vi "Initialization Error Status.vi"(8 "error in (no error)":errorcluster, 11 "Node Ptr":T1 format="%.0x") -> (0 "error out":errorcluster)   [LabVIEW 2015, in "DMM-SWITCH-ScanList System Explorer.lvlib"]
uses:
  DMM-SWITCH-ScanList System Explorer.lvlib
  <vilib>/NI Veristand/Custom Device API/Custom Device Item Ref.ctl
  <vilib>/NI Veristand/Custom Device API/Custom Device API.lvlib
panel:
  out "Channel Settings":i32(listbox)
  in  "Header":cluster{"Section Name":string}={"Section Name"="Custom Device Item Settings"}
  in  "Description":string
  in  "Name":string
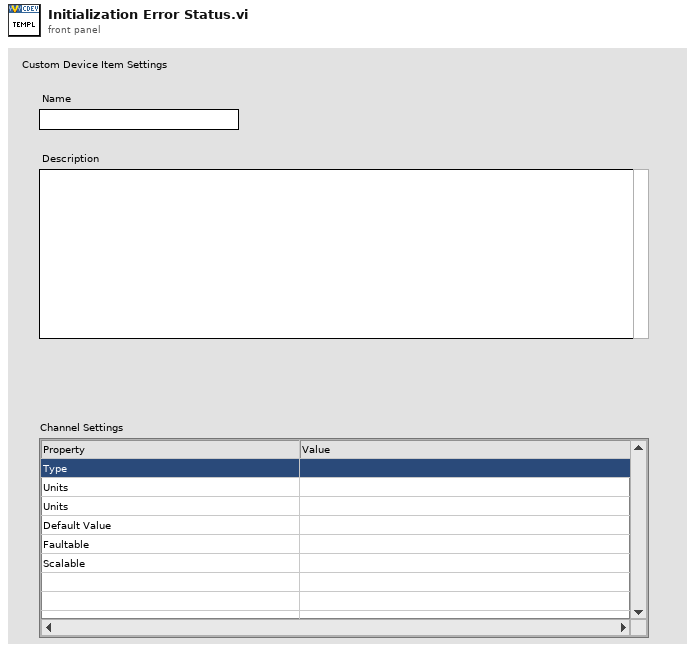
[diagram p1: front panel]
types:
  T1 = typedef "Custom Device API.lvlib/Custom Device Item Ref.ctl" = u64
  T2 = typedef "Custom Device API.lvlib/Custom Device Item Info.ctl" = cluster{"Name":string, "Is Channel":bool, "GUID":string, "Is Waveform":bool}
  T3 = typedef "Custom Device API.lvlib/Custom Device Commands.ctl" = enum16{"Default", "Item renamed", "Shutdown", "Dynamic button pressed"}
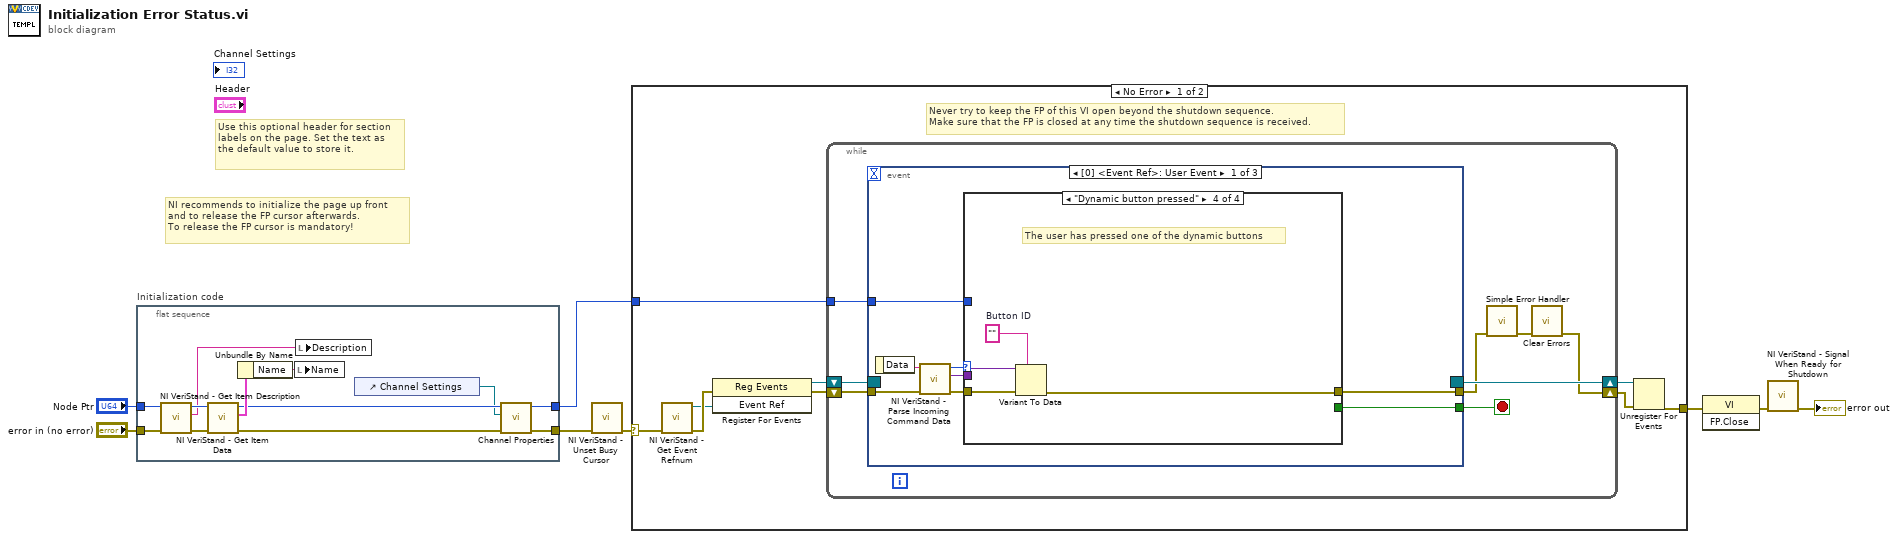
[diagram p0: block diagram]
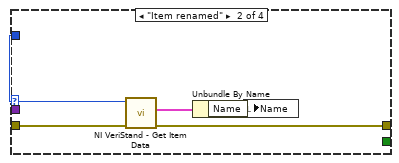
[diagram p3: hidden frame]
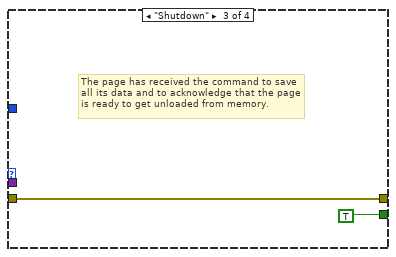
[diagram p4: hidden frame]
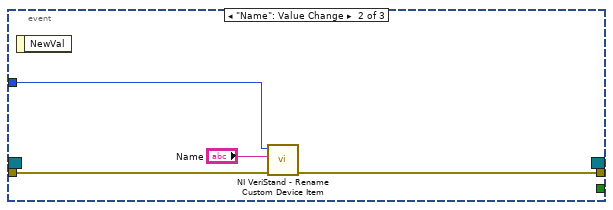
[diagram p5: hidden frame]
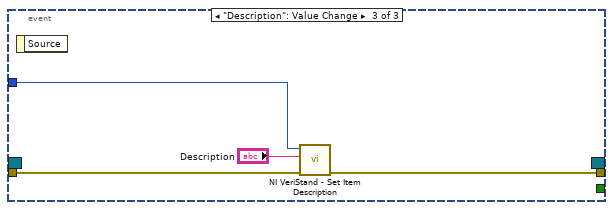
[diagram p6: hidden frame]
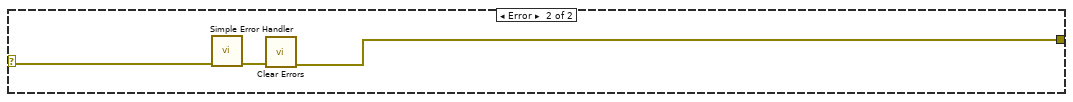
[diagram p7: hidden frame]
diagram:
  # "Use this optional header for section labels on the page. Set the text as the default value to store it."
  # "NI recommends to initialize the page up front\nand to release the FP cursor afterwards.\nTo release the FP cursor is mandatory!"
  n1 = flat-sequence "Initialization code" {
    tunnel: "error in (no error)" -> [w19]
    tunnel: "Node Ptr" -> [w18]
    tunnel: [w10] -> w4
    tunnel: [w11] -> w1
    frame #0 {
      n2 = call <vilib>:"NI VeriStand - Get Item Description.vi"("error in (no error)"=w19, "Item Ref in"=w18) -> ("error out"=w16:errorcluster, "Description"=w17:string, "Item Ref out"=w20:T1)  [unwired: 7 out]
      n3 = call <vilib>:"NI VeriStand - Get Item Data.vi"("error in (no error)"=w16, "Item Ref in"=w20) -> ("error out"=w12:errorcluster, "Item Info"=w15:T2, "Item Ref out"=w13:T1)  [unwired: 7 out]
      n4 = Unbundle By Name(w15) -> ("Name"=w14:string)
      n5 = local write "Name"(w14) -> ()
      n6 = local write "Description"(w17) -> ()
      n7 = control-ref of="Channel Settings"() -> (w9:refnum<vi>)
      n8 = call "Channel Properties.vi"("error in (no error)"=w12, "Channel Settings Ref In"=w9, "Channel Ref In"=w13) -> ("error out"=w10:errorcluster, "Channel Ref Out"=w11:T1)  [unwired: 7 in]
    }
  }
  n9 = call <vilib>:"NI VeriStand - Unset Busy Cursor.vi"("error in (no error)"=w4) -> ("error out"=w3:errorcluster)  [unwired: 10 out]
  n10 = case shown="No Error" w3 {
    selector: w3 -> [w21 w68]
    tunnel: [w26 w66] -> w8
    tunnel: w1 -> [w22 _]
    frame No Error {
      # "Never try to keep the FP of this VI open beyond the shutdown sequence.\nMake sure that the FP is closed at any time the shutdown sequence is received."
      n11 = call <vilib>:"NI VeriStand - Get Event Refnum.vi"("error in (no error)"=w21) -> ("error out"=w29:errorcluster, "Event Ref"=w25:refnum<user-event>)  [unwired: 9 out]
      n12 = register-events(error in=w29, w25) -> (reference out=w23:refnum<event-registration>, error out=w24:errorcluster)  [unwired: 1 in]
      n13 = while {
        tunnel: w22 -> [w33]
        shift-right: [w30] -> w27
        shift-left: w24 -> [w36]
        shift-right: [w37] -> w28
        shift-left: w23 -> [w35]
        stop <- w34 stop-if-true
        n14 = event shown="[0] <Event Ref>: User Event" {
          selector: w35 -> [_ _ _]
          dyn-events: [_ _ _] -> w37
          timeout: _ -> [_ _ _]
          tunnel: w36 -> [w45 w61 w64]
          tunnel: [w41 _ _] -> w34
          tunnel: [w40 w60 w63] -> w32
          tunnel: w33 -> [w39 w59 w65]
          event User Event {
            n15 = event-data() -> ("Data"=w44:string)  [unwired: 1 out]
            n16 = call <vilib>:"NI VeriStand - Parse Incoming Command Data.vi"("error in (no error)"=w45, "Incoming data"=w44) -> ("error out"=w43:errorcluster, "Outgoing data"=w38:variant, "Action"=w42:T3)  [unwired: 7 out]
            n17 = case shown="\"Dynamic button pressed\"" w42 {
              tunnel: w43 -> [w46 w51 w52 w57]
              tunnel: [_ _ TRUE _] -> w41
              tunnel: [w46 w48 w52 w54] -> w40
              tunnel: w39 -> [_ w50 _ _]
              tunnel: w38 -> [_ _ _ w56]
              frame "Default", Default {
              }
              frame "Item renamed" {
                n18 = call <vilib>:"NI VeriStand - Get Item Data.vi"("error in (no error)"=w51, "Item Ref in"=w50) -> ("error out"=w48:errorcluster, "Item Info"=w49:T2)  [unwired: 8 out]
                n19 = Unbundle By Name(w49) -> ("Name"=w47:string)
                n20 = local write "Name"(w47) -> ()
              }
              frame "Shutdown" {
                # "The page has received the command to save all its data and to acknowledge that the page is ready to get unloaded from memory."
              }
              frame "Dynamic button pressed" {
                w55 = ""  # Button ID
                # "The user has pressed one of the dynamic buttons"
                n21 = Variant To Data(error in=w57, type=w55, Variant=w56) -> (error out=w54:errorcluster)  [unwired: 1 out]
              }
            }
          }
          event "Name": Value Change {
            n22 = event-data() -> ()  [unwired: 2 out]
            n23 = call <vilib>:"NI VeriStand - Rename Custom Device Item.vi"("error in (no error)"=w61, "New Name"="Name", "Item Ref in"=w59) -> ("error out"=w60:errorcluster)  [unwired: 1 in, 7 out]
          }
          event "Description": Value Change {
            n24 = event-data() -> ()  [unwired: 2 out]
            n25 = call <vilib>:"NI VeriStand - Set Item Description.vi"("error in (no error)"=w64, "Description"="Description", "Item Ref in"=w65) -> ("error out"=w63:errorcluster)  [unwired: 8 out]
          }
        }
        n26 = call <vilib>:"Simple Error Handler.vi"("error in (no error)"=w32) -> ("error out"=w31:errorcluster)  [unwired: 1 in, 7 out]
        n27 = call <vilib>:"Clear Errors.vi"("error in (no error)"=w31) -> ("error out"=w30:errorcluster)  [unwired: 1 in, 5 out]
      }
      n28 = Unregister For Events(event registration refnum=w28, error in=w27) -> (error out=w26:errorcluster)
    }
    frame Error {
      n29 = call <vilib>:"Simple Error Handler.vi"("error in (no error)"=w68) -> ("error out"=w67:errorcluster)  [unwired: 1 in, 7 out]
      n30 = call <vilib>:"Clear Errors.vi"("error in (no error)"=w67) -> ("error out"=w66:errorcluster)  [unwired: 1 in, 5 out]
    }
  }
  n31 = invoke class="VI" method="FP.Close"(error in=w8) -> (error out=w7:errorcluster)  [unwired: 2 in, 2 out]
  n32 = call <vilib>:"NI VeriStand - Signal When Ready for Shutdown.vi"("error in (no error)"=w7) -> ("error out"=→"error out":errorcluster)  [unwired: 10 out]
